vi "Vector Field.vi"() -> ()   [LabVIEW 2020]
uses:
  <vilib>/Utility/sysdir.llb/System Directory Type.ctl
  <instrlib>/tio-labview/TIO Library/TIO Stream Open.vi
  <instrlib>/tio-labview/TIO Library/TIO RPC Send REQuest.vi
  <instrlib>/tio-labview/Labview Signal Processing/Log Binning.vi
  <vilib>/Utility/error.llb/Clear Errors.vi
  <instrlib>/tio-labview/TIO Library/TIO RPC Parse Reply.vi
  <instrlib>/tio-labview/TIO Library/TIO RPC Parse Reply Error.vi
  <instrlib>/tio-labview/TIO Library/TIO Data Stream Parse timebase Info.vi
  <instrlib>/tio-labview/TIO Library/TIO Data Stream Parse pstream Info.vi
  <instrlib>/tio-labview/TIO Library/TIO Data Stream Parse dstream Info.vi
  <vilib>/Utility/High Resolution Relative Seconds.vi
  <instrlib>/tio-labview/TIO Library/TIO Serial Port Name Search.vi
  <instrlib>/tio-labview/TIO Library/TIO Stream Write.vi
  <instrlib>/tio-labview/TIO Library/TIO RPC Form Request.vi
  <instrlib>/tio-labview/Labview Signal Processing/Log Range.vi
  <instrlib>/tio-labview/TIO Library/TIO SLIP Serial Write.vi
  <instrlib>/tio-labview/TIO Library/TIO Form Packet.vi
  <instrlib>/tio-labview/TIO Library/TIO SLIP Encode.vi
  <instrlib>/tio-labview/TIO Library/TIO Serial Checksum CRC32.vi
  <vilib>/Utility/tcp.llb/UDP Multicast Open.vi
  <vilib>/Utility/tcp.llb/UDP Multicast Read-Write Open.vi
  <instrlib>/tio-labview/TIO Library/TIO Serial Port Discovery.vi
  <vilib>/Instr/_visa.llb/VISA Configure Serial Port (Instr).vi
  <instrlib>/tio-labview/TIO Library/TIO RPC Blocking.vi
  <vilib>/Analysis/6fits.llb/General Polynomial Fit.vi
  <vilib>/measure/maspectr.llb/FFT Power Spectrum and PSD.vi
  <vilib>/measure/maspectr.llb/FFT Power Spectrum and PSD for 1 Chan.vi
  <instrlib>/tio-labview/TIO Library/TIO Stream Read Non-blocking.vi
  <instrlib>/tio-labview/TIO Library/TIO RPC Send Heartbeat.vi
panel:
  in  "Enable Y":bool caption="Auto Cal"
  in  "Enable X":bool caption="Auto Cal"
  in  "Bin":bool=TRUE
  in  "Clear A":bool
  in  "Save A":bool
  in  "Log?":bool
  in  "Path":path
  in  "Auto Cal":bool
  in  "Auto Zero":bool
  in  "Quit":bool
  in  "Reset":bool
  in  "Duration":dbl[unit]=100.0
  in  "URL":refnum<visa-resource-name>="tcp://localhost"
  out "ID":string
  out "Timeseries":cluster{"start":dbl, "dt":dbl, dbl[][]}(graph)
  out "Noise":T1(graph)
  # "Vector Field"
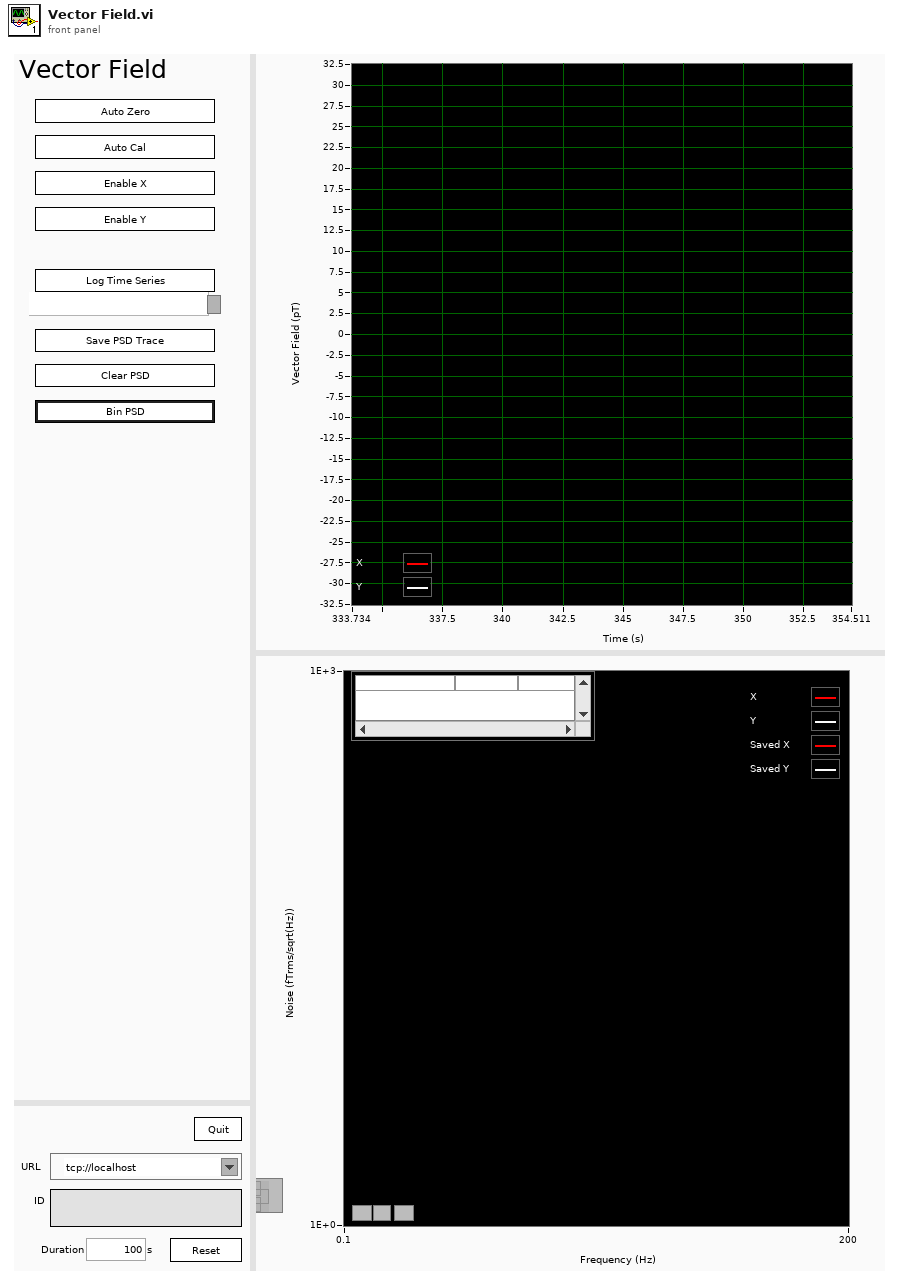
[diagram p1: front panel]
types:
  T1 = cluster{"Frequencies Binned":dbl[], "Spectrum Binned":dbl[]}[]
  T2 = typedef "System Directory Type.ctl" = i32
  T3 = cluster{"TS Connection":cluster{"Type":enum16{"Serial", "TCP", "UDP", "mUDP"}, "URL":refnum<visa-resource-name>, "TO":u32, "Addr":u32, "Port":i32, "TCP":refnum<k5>, "UDP":refnum<k16>, "Route":string}, "REQ":refnum<queue>, "REP":refnum<queue>}
  T4 = cluster{"Frequencies Binned":dbl[], "Spectrum Binned":dbl[]}
  T5 = cluster{"Awaiting REP":bool, "REQ ID":u32, "streams in":cluster{"id":u16, "timebase id":u16, "period":u32, "offset":u32, "sample number":u64, "total components":u16, "flags":u16, "components":cluster{"source id":u16, "flags":u16, "period":u32, "offset":u32}[]}[], "sources":cluster{"id":u16, "timebase_id":u16, "period":u32, "offset":u32, "fmt":i32, "flags":u16, "channels":u16, "type":u8, "name":string, "column names":string[], "title":string, "units":string}[], "timebases":cluster{"id":u16, "source":u8, "epoch":u8, "start time":u64, "period numerator (µs)":u32, "period denominator (µs)":u32, "flags":u32, "stability":sgl, "source id":string}[]}
  T6 = cluster{"stream ID":u16, "Sample Number":u32, "Raw Data":string}
  T7 = cluster{"TC Connection":cluster{"Type":enum16{"Serial", "TCP", "UDP", "mUDP"}, "URL":refnum<visa-resource-name>, "TO":u32, "Addr":u32, "Port":i32, "TCP":refnum<k5>, "UDP":refnum<k16>, "Route":string}, "REQ":refnum<queue>, "REP":refnum<queue>}
  T8 = cluster{"Name":string, "Waveform":cluster{"start":dbl, "dt":dbl, "Timeseries":dbl[][]}}[]
  T9 = cluster{"start":dbl, "dt":dbl, "Timeseries":dbl[][]}
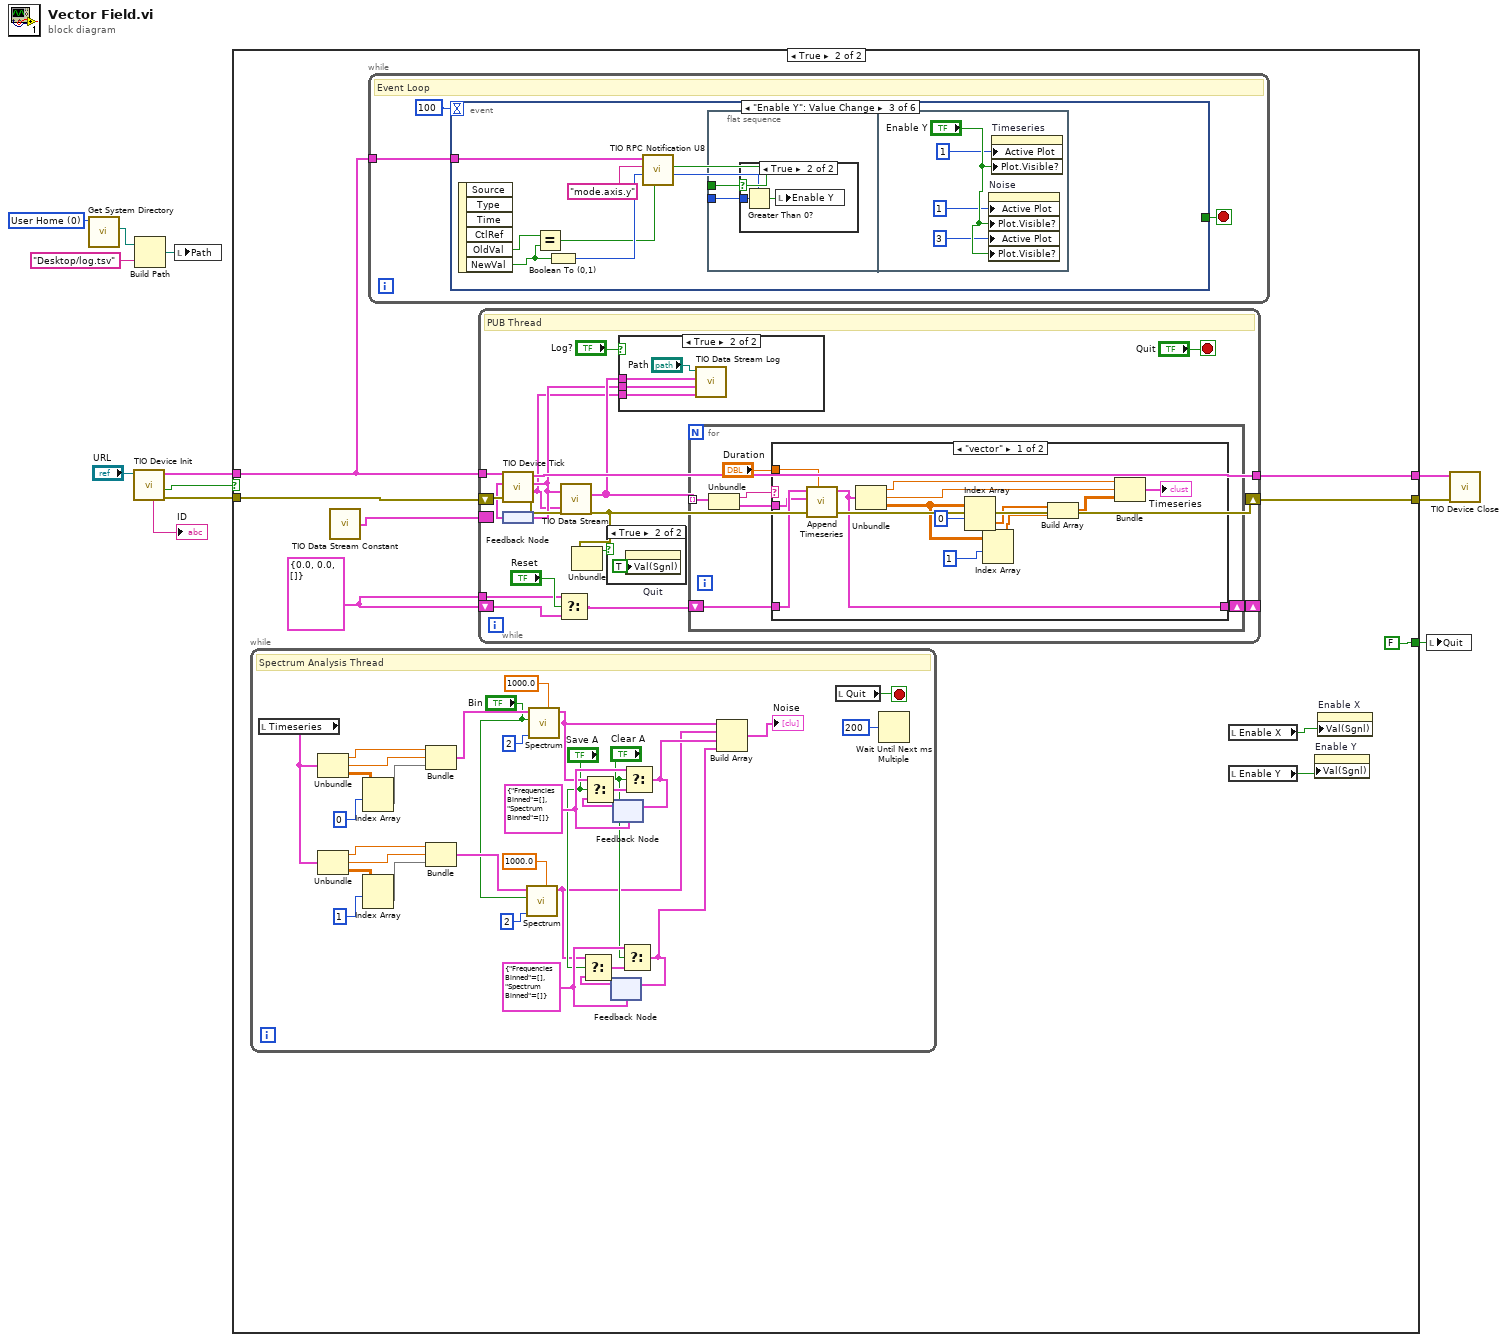
[diagram p0: block diagram]
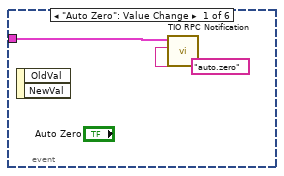
[diagram p6: hidden frame]
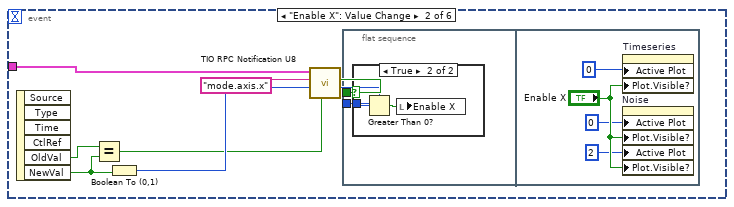
[diagram p7: hidden frame]
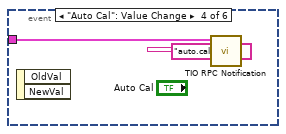
[diagram p10: hidden frame]
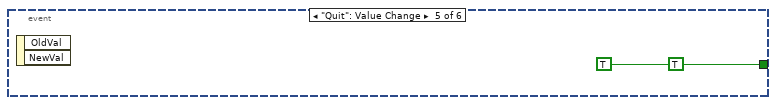
[diagram p11: hidden frame]
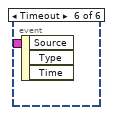
[diagram p12: hidden frame]
diagram:
  w1 = T2 0 items=["User Home"=0, "User Desktop"=1, "User Documents"=2, "User Application Data"=3, "User Preferences"=4, "User Temporary"=5, "Public Documents"=6, "Public Application Data"=7, "Public Preferences"=8, "Public Cache"=13, "System Core Libraries"=9, "System Installed Libraries"=10, "Application Files"=11, "Boot Volume Root"=12] ("system directory type")
  n1 = call <vilib>:"Get System Directory.vi"("system directory type"=w1) -> ("system directory"=w4:path)  [unwired: 10 in]
  n2 = call <instrlib>:"TIO Device Init.vi"("URL"="URL") -> ("error out"=w9:errorcluster, "Connected"=w11:bool, "TIO"=w8:T3, "ID Verified"=→"ID":string)  [unwired: 6 in, 1 out]
  n3 = Build Path(base path=w4, name or relative path="Desktop/log.tsv") -> (appended path=w2:path)
  n4 = local write "Path"(w2) -> ()
  n5 = case shown="True" w11 {
    tunnel: w8 -> [w14 w17]
    tunnel: [_ FALSE ("Quit")] -> w10
    tunnel: w9 -> [w13 w18]
    tunnel: [w13 w20] -> w7
    tunnel: [w14 w19] -> w6
    frame False {
    }
    frame True {
      w23 = cluster{dbl, dbl, dbl[][]} {0.0, 0.0, []} ("Waveform Timeseries")
      n6 = while {
        stop <- w53 stop-if-true
        w38 = T4 {"Frequencies Binned"=[], "Spectrum Binned"=[]} ("Cluster")
        w50 = T4 {"Frequencies Binned"=[], "Spectrum Binned"=[]} ("Cluster")
        # "Spectrum Analysis Thread"
        n7 = local read "Timeseries"() -> (w30:cluster{"start":dbl, "dt":dbl, dbl[][]})
        n8 = Unbundle(w30) -> ("start"=w46:dbl, "dt"=w45:dbl, w48:dbl[][])
        n9 = Unbundle(w30) -> ("start"=w33:dbl, "dt"=w34:dbl, w31:dbl[][])
        n10 = Index Array(array=w48, index (row)=0) -> (element=w44:dbl[])  [unwired: 1 in]
        n11 = Index Array(array=w31, index (row)=1) -> (element=w35:dbl[])  [unwired: 1 in]
        n12 = Bundle("start"=w46, "dt"=w45, w44) -> (w43:cluster{"start":dbl, "dt":dbl, dbl[]})  [unwired: 1 in]
        n13 = Bundle("start"=w33, "dt"=w34, w35) -> (w29:cluster{"start":dbl, "dt":dbl, dbl[]})  [unwired: 1 in]
        n14 = call <instrlib>:"Spectrum.vi"("Gain"=1000.0, "Remove Polynomial Order"=2, "Binning"="Bin", "Waveform 1"=w29) -> ("Cluster"=w25:T4)  [unwired: 5 in]
        n15 = call <instrlib>:"Spectrum.vi"("Gain"=1000.0, "Remove Polynomial Order"=2, "Binning"="Bin", "Waveform 1"=w43) -> ("Cluster"=w49:T4)  [unwired: 5 in]
        n16 = feedback #1(w38) -> (w39:T4)
        n17 = Select(t=w25, s="Save A", f=w39) -> (s? t:f=w40:T4)
        n18 = feedback #2(w50) -> (w51:T4)
        n19 = Select(t=w49, s="Save A", f=w51) -> (s? t:f=w52:T4)
        n20 = Select(t=w38, s="Clear A", f=w40) -> (s? t:f=w28:T4)
        n21 = feedback-in #1(w28) -> ()
        n22 = Select(t=w50, s="Clear A", f=w52) -> (s? t:f=w26:T4)
        n23 = feedback-in #2(w26) -> ()
        n24 = Build Array(w49, w25, w26, w28) -> (→"Noise":T1)
        n25 = local read "Quit"() -> (w53:bool)
        n26 = Wait Until Next ms Multiple(millisecond multiple=u32 200) -> ()  [unwired: 1 out]
      }
      n27 = call <instrlib>:"TIO Data Stream Constant.vi"() -> ("TIO State"=w21:T5)
      n28 = while {
        tunnel: w17 -> [w99]
        stop <- w98 stop-if-true
        # "Event Loop"
        n29 = event shown="[2] \"Enable Y\": Value Change" {
          selector: _ -> [_ _ _ _ _ _]
          dyn-events: _ -> [_ _ _ _ _ _]
          timeout: 100 -> [_ _ _ _ _ _]
          tunnel: w99 -> [w102 w109 w125 w136 _ _]
          tunnel: [_ _ _ _ TRUE ("Quit") _] -> w98
          event "Auto Zero": Value Change {
            n30 = event-data() -> ()  [unwired: 1 in, 2 out]
            n31 = call <instrlib>:"TIO RPC Notification.vi"("Topic"="auto.zero", "TIO"=w102) -> ()  [unwired: 6 in, 3 out]
          }
          event "Enable X": Value Change {
            n32 = event-data() -> ("OldVal"=w107:bool, "NewVal"=w106:bool)  [unwired: 1 in, 4 out]
            n33 = Equal?(x=w107, y=w106) -> (x = y?=w103:bool)
            n34 = Boolean To (0,1)(Boolean=w106) -> (0, 1=w108:i16)
            n35 = call <instrlib>:"TIO RPC Notification U8.vi"("Read"=w103, "U8"=w108, "Topic"="mode.axis.x", "TIO"=w109) -> ("U8"=w104:u8, "Response"=w105:bool)  [unwired: 4 in, 1 out]
            n36 = flat-sequence {
              tunnel: w105 -> [w112]
              tunnel: w104 -> [w111]
              frame #0 {
                n37 = case shown="True" w112 {
                  tunnel: w111 -> [_ w114]
                  frame False {
                  }
                  frame True {
                    n38 = Greater Than 0?(x=w114) -> (x > 0?=w113:bool)
                    n39 = local write "Enable X"(w113) -> ()
                  }
                }
              }
              frame #1 {
                n40 = property on="Timeseries" class="WFGraph (strict)"("Active Plot"=u32 0, "Plot.Visible?"="Enable X") -> ()  [unwired: 2 in, 2 out]
                n41 = property on="Noise" class="XYGraph (strict)"("Active Plot"=u32 0, "Plot.Visible?"="Enable X", "Active Plot"=u32 2, "Plot.Visible?"="Enable X") -> ()  [unwired: 2 in, 2 out]
              }
            }
          }
          event "Enable Y": Value Change {
            n42 = event-data() -> ("OldVal"=w122:bool, "NewVal"=w123:bool)  [unwired: 1 in, 4 out]
            n43 = Equal?(x=w122, y=w123) -> (x = y?=w119:bool)
            n44 = Boolean To (0,1)(Boolean=w123) -> (0, 1=w124:i16)
            n45 = call <instrlib>:"TIO RPC Notification U8.vi"("Read"=w119, "U8"=w124, "Topic"="mode.axis.y", "TIO"=w125) -> ("U8"=w120:u8, "Response"=w121:bool)  [unwired: 4 in, 1 out]
            n46 = flat-sequence {
              tunnel: w121 -> [w128]
              tunnel: w120 -> [w127]
              frame #0 {
                n47 = case shown="True" w128 {
                  tunnel: w127 -> [_ w130]
                  frame False {
                  }
                  frame True {
                    n48 = Greater Than 0?(x=w130) -> (x > 0?=w129:bool)
                    n49 = local write "Enable Y"(w129) -> ()
                  }
                }
              }
              frame #1 {
                n50 = property on="Noise" class="XYGraph (strict)"("Active Plot"=u32 1, "Plot.Visible?"="Enable Y", "Active Plot"=u32 3, "Plot.Visible?"="Enable Y") -> ()  [unwired: 2 in, 2 out]
                n51 = property on="Timeseries" class="WFGraph (strict)"("Active Plot"=u32 1, "Plot.Visible?"="Enable Y") -> ()  [unwired: 2 in, 2 out]
              }
            }
          }
          event "Auto Cal": Value Change {
            n52 = event-data() -> ()  [unwired: 1 in, 2 out]
            n53 = call <instrlib>:"TIO RPC Notification.vi"("Topic"="auto.calibrate", "TIO"=w136) -> ()  [unwired: 6 in, 3 out]
          }
          event "Quit": Value Change {
            (unwired) TRUE ("Quit")
            n54 = event-data() -> ()  [unwired: 1 in, 2 out]
          }
          event Timeout {
            n55 = event-data() -> ()  [unwired: 1 in, 3 out]
          }
        }
      }
      n56 = while {
        shift-right: [w72] -> _
        shift-left: w23 -> [w70]
        tunnel: w23 -> [w68]
        tunnel: w17 -> [w65]
        border: w21 -> [_]
        tunnel: [w63] -> w19
        shift-right: [w60] -> w20
        shift-left: w18 -> [w66]
        stop <- "Quit" stop-if-true
        # "PUB Thread"
        n57 = feedback #3() -> (w64:T5)
        n58 = call <instrlib>:"TIO Device Tick.vi"("Error in"=w66, "TIO State"=w64, "TIO"=w65) -> ("Error out"=w60:errorcluster, "Data Out"=w57:T6, "TIO State"=w58:T5, "TIO"=w63:T7)  [unwired: 5 in]
        n59 = feedback-in #3(w58) -> ()
        n60 = Select(t=w68, s="Reset", f=w70) -> (s? t:f=w69:cluster{dbl, dbl, dbl[][]})
        n61 = call <instrlib>:"TIO Data Stream.vi"("Raw Data"=w57, "TIO State"=w58) -> ("Data Out"=w59:T8)
        n62 = Unbundle(w60) -> ("status"=w62:bool)  [unwired: 2 out]
        n63 = case shown="True" w62 {
          frame False {
          }
          frame True {
            n64 = property on="Quit" class="Bool (strict)"("Val(Sgnl)"=TRUE ("Value (Signaling)")) -> ()  [unwired: 2 in, 2 out]
          }
        }
        n65 = case shown="True" "Log?" {
          tunnel: w59 -> [_ w73]
          tunnel: w58 -> [_ w76]
          tunnel: w57 -> [_ w75]
          frame False {
          }
          frame True {
            n66 = call <instrlib>:"TIO Data Stream Log.vi"(8:"Data Out"=w75, "TIO State"=w76, 10:"Data Out"=w73, "Log to file"="Path") -> ()  [unwired: 8 in]
          }
        }
        n67 = for {
          shift-right: [w83] -> w72
          shift-left: w69 -> [w82]
          tunnel: w59 -> [w80] mode=indexing
          n68 = Unbundle(w80) -> ("Name"=w78:string, "Waveform"=w79:T9)
          n69 = case shown="\"vector\"" w78 {
            tunnel: "Duration" -> [w96 _]
            tunnel: [w95 w97] -> w83
            tunnel: w82 -> [w94 w97]
            tunnel: w79 -> [w93 _]
            frame "vector" {
              n70 = call <instrlib>:"Append Timeseries.vi"("Duration"=w96, "In New"=w93, "In Old"=w94) -> ("Appended"=w95:T9)  [unwired: 8 in]
              n71 = Unbundle(w95) -> ("start"=w91:dbl, "dt"=w90:dbl, "Timeseries"=w92:dbl[][])
              n72 = Index Array(array=w92, index (row)=0) -> (element=w89:dbl[])  [unwired: 1 in]
              n73 = Index Array(array=w92, index (row)=1) -> (element=w88:dbl[])  [unwired: 1 in]
              n74 = Build Array(w89, w88) -> (w87:dbl[][])
              n75 = Bundle("start"=w91, "dt"=w90, w87) -> (→"Timeseries":cluster{"start":dbl, "dt":dbl, dbl[][]})  [unwired: 1 in]
            }
            frame Default {
            }
          }
        }
      }
      n76 = local read "Enable X"() -> (w16:bool)
      n77 = local read "Enable Y"() -> (w15:bool)
      n78 = property on="Enable Y" class="Bool (strict)"("Val(Sgnl)"=w15) -> ()  [unwired: 2 in, 2 out]
      n79 = property on="Enable X" class="Bool (strict)"("Val(Sgnl)"=w16) -> ()  [unwired: 2 in, 2 out]
    }
  }
  n80 = local write "Quit"(w10) -> ()
  n81 = call <instrlib>:"TIO Device Close.vi"("Error in"=w7, "TIO"=w6) -> ()  [unwired: 10 in]
